vi "ReadFits-ExtractROI.vi"() -> ()   [LabVIEW 2011]
uses:
  <vilib>/Analysis/6fits.llb/Curve Fitting Criteria.ctl
  gfitsio/gfitsio-read-image-subset-i32-2d.vi
  Polymorphics/Distance(single).vi
  gfitsio/gfitsio.lvlib
  <vilib>/Analysis/NI_AALBase.lvlib
  <vilib>/Analysis/NI_AALPro.lvlib
panel:
  out "residue":dbl
  out "stdv":dbl
  out "amplitude":dbl
  out "center":dbl
  out "offset":dbl
  out "TmpData":i32[][](array[numeric])
  out "PSF X":dbl[](array[numeric])
  out "PSF Y":dbl[](array[numeric])
  in  "Use Barycen ?":bool
  out "XY Graph":cluster{"PSF X":dbl[], "PSF Y":dbl[]}[](graph)
  out "Cen Y":dbl
  out "Cen X":dbl
  out "ImageMedian":dbl format="%0.2f"
  out "Histogram Graph":T1(graph)
  in  "process":bool
  out "OutskirtMedian":dbl format="%0.2f"
  in  "save":bool
  in  "Length Y":i32
  in  "Length X":i32
  in  "Start Y":i32
  in  "Start X":i32
  out "ROI":i32[][](graph)
  out "Full Fits":i32[][](graph)
  in  "Path":path
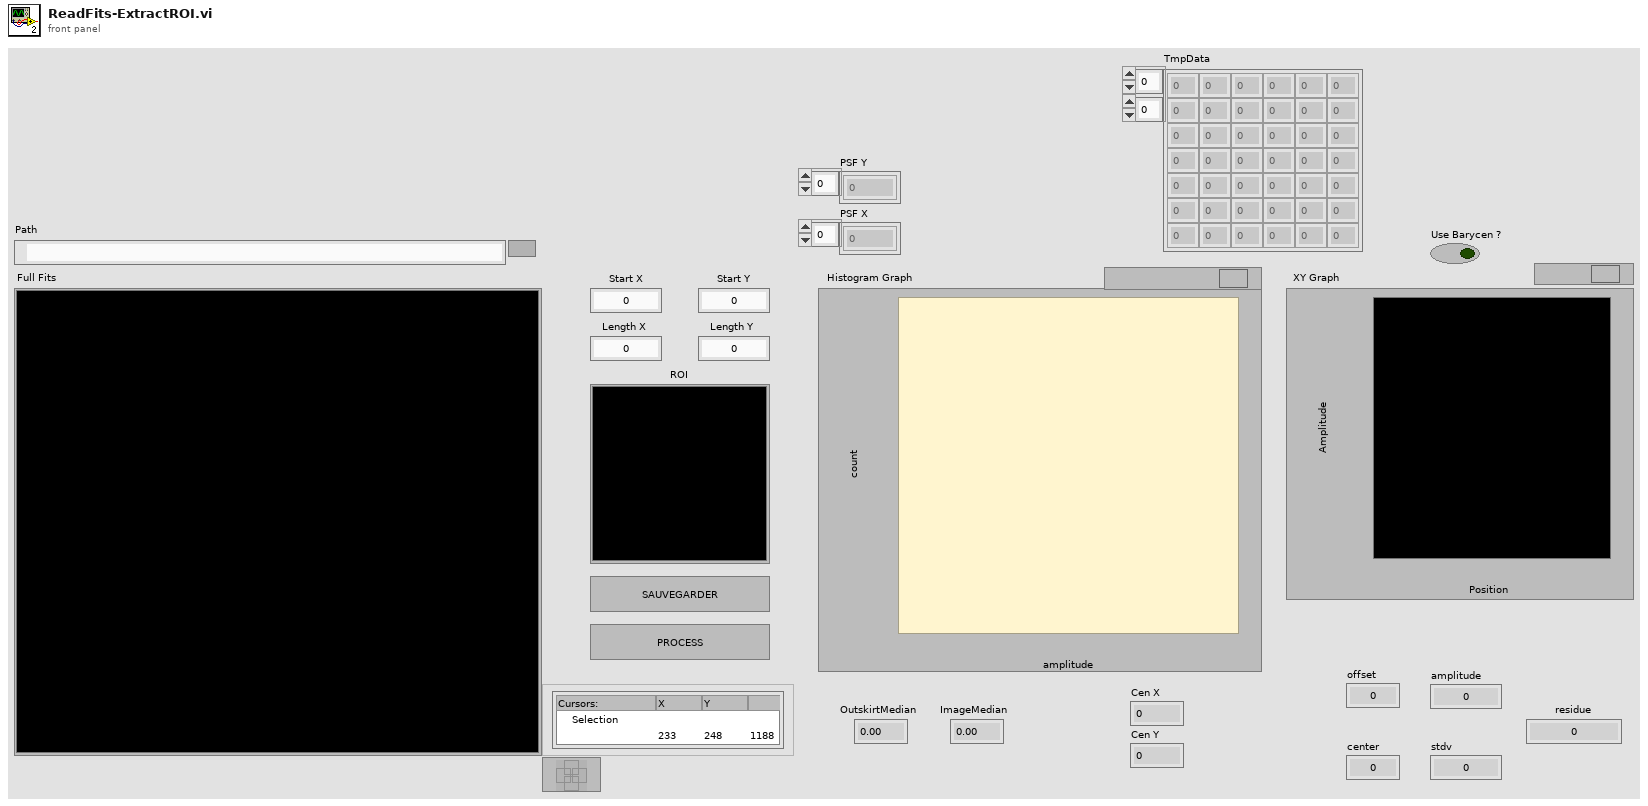
[diagram p1: front panel]
types:
  T1 = cluster{"X Values":dbl[], "Histogram: h(x)":i32[]}
  T2 = cluster{"amp min":dbl, "amp max":dbl, "center min":dbl, "center max":dbl, "deviation min":dbl, "deviation max":dbl, "offset min":dbl, "offset max":dbl}
  T3 = typedef "gfitsio.lvlib/gfitsio-refnum.ctl" = refnum<k1>
  T4 = typedef "NI_AALPro.lvlib/Curve Fitting Criteria.ctl" = u16
  T5 = cluster{dbl, "center min":dbl, "center min":dbl, "center min":dbl}
  T6 = cluster{"PSF X":dbl[], "Best Gaussian Fit":dbl[]}
  T7 = cluster{"PSF X":dbl[], "Best Gaussian Fit":dbl[]}[]
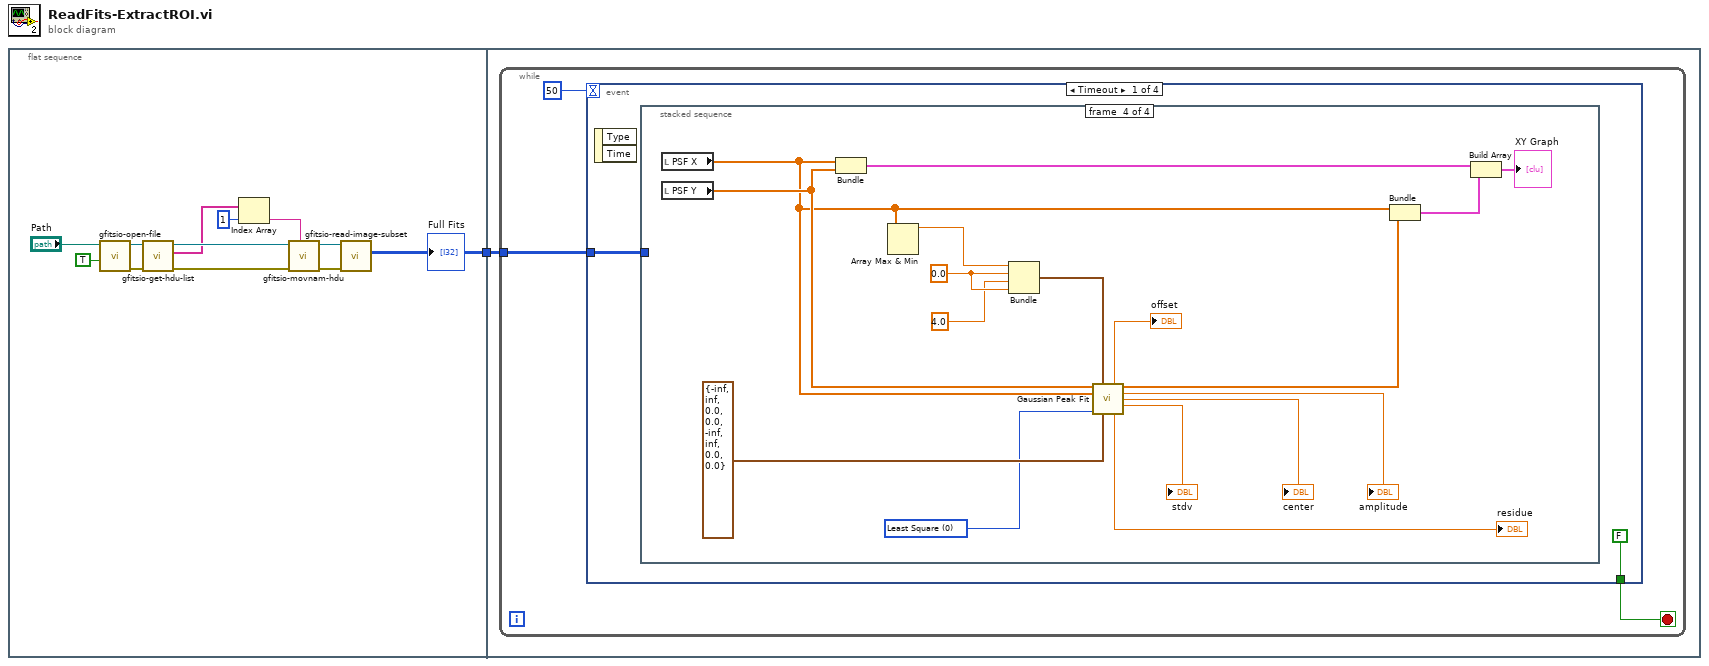
[diagram p0: block diagram]
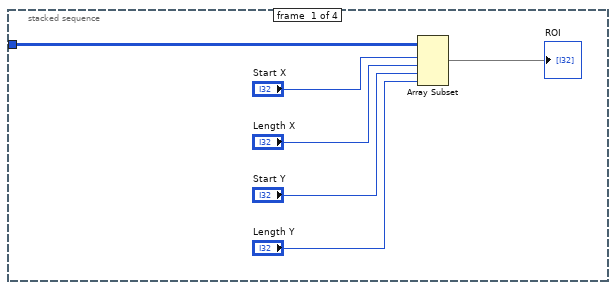
[diagram p2: hidden frame]
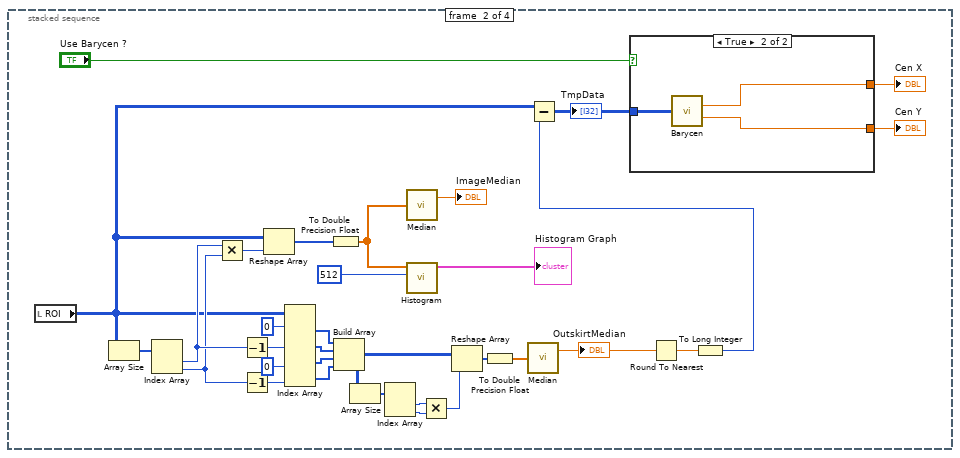
[diagram p3: hidden frame]
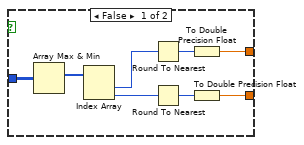
[diagram p4: hidden frame]
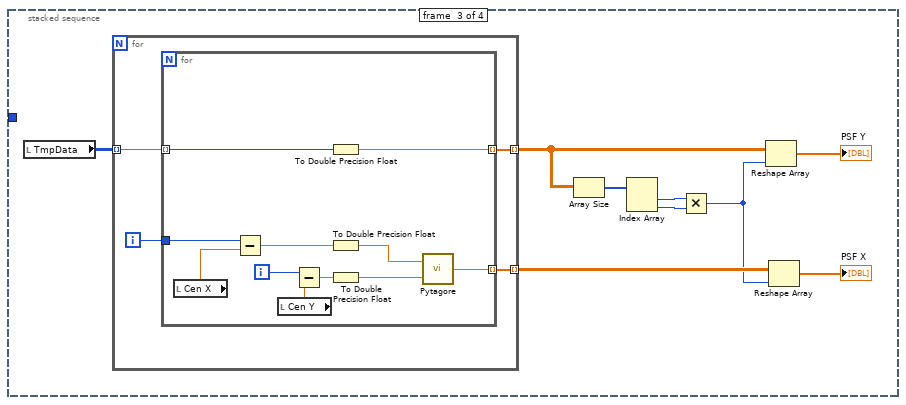
[diagram p5: hidden frame]
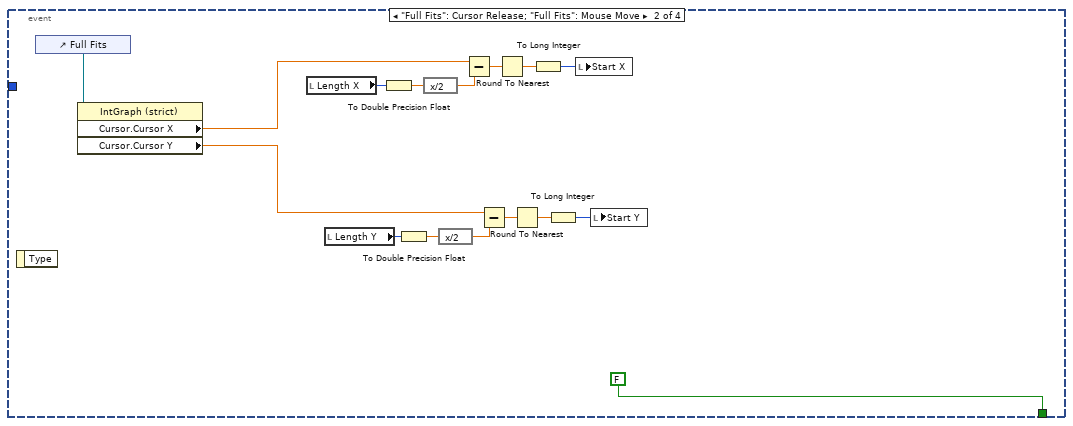
[diagram p6: hidden frame]
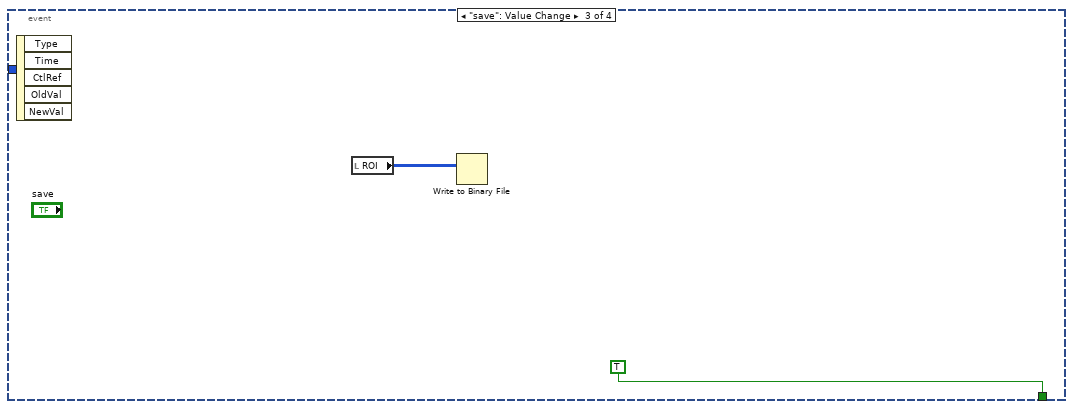
[diagram p7: hidden frame]
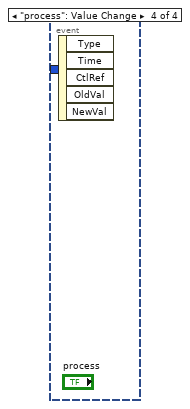
[diagram p8: hidden frame]
diagram:
  n1 = flat-sequence {
    tunnel: [w2] -> w1
    tunnel: w1 -> [w14]
    frame #0 {
      n2 = call "gfitsio-open-file.vi"("read only? (T:no)"=TRUE, "path"="Path") -> ("error out"=w6:errorcluster, "gfits refnum"=w7:T3)  [unwired: 8 in]
      n3 = call "gfitsio-get-hdu-list.vi"("error in (no error)"=w6, "gfits refnum"=w7) -> ("error out"=w8:errorcluster, "hdu names"=w5:string[], "dup gfits refnum"=w9:T3)  [unwired: 6 in, 1 out]
      n4 = Index Array(array=w5, index=1) -> (element=w3:string)
      n5 = call "gfitsio-movnam-hdu.vi"("extname"=w3, "error in (no error)"=w8, "gfits refnum"=w9) -> ("error out"=w11:errorcluster, "dup gfits refnum"=w10:T3)  [unwired: 7 in]
      n6 = call-poly "gfitsio-read-image-subset.vi"("error in (no error)"=w11, "gfits refnum"=w10) -> ("data"=w2:i32[][])  [unwired: 6 in, 3 out]
      "Full Fits" <- w2
    }
    frame #1 {
      n7 = while {
        tunnel: w14 -> [w17]
        stop <- w15 stop-if-true
        n8 = event shown="[0] Timeout" {
          selector: _ -> [_ _ _ _]
          dyn-events: _ -> [_ _ _ _]
          timeout: 50 -> [_ _ _ _]
          tunnel: w17 -> [w19 _ _ _]
          tunnel: [FALSE FALSE TRUE _] -> w15
          event Timeout {
            n9 = event-data() -> ()  [unwired: 1 in, 2 out]
            n10 = stacked-sequence {
              tunnel: w19 -> [w25 _ _ _]
              frame #0 {
                n11 = Array Subset(array=w25, index (row)="Start X", length (row)="Length X", index (col)="Start Y", length (col)="Length Y") -> (→"ROI":i32[][])
              }
              frame #1 {
                n12 = local read "ROI"() -> (w27:i32[][])
                n13 = Array Size(array=w27) -> (size(s)=w57:i32[])
                n14 = Index Array(array=w57) -> (element #1=w40:i32, element #2=w39:i32)  [unwired: 2 in]
                n15 = Multiply(x=w40, y=w39) -> (x*y=w41:i32)
                n16 = Decrement(x=w40) -> (x-1=w55:i32)
                n17 = Decrement(x=w39) -> (x-1=w54:i32)
                n18 = Reshape Array(w27, w41) -> (w38:i32[])
                n19 = Index Array(array=w27, index (row) #1=0, index (row) #2=w55, index (col) #3=0, index (col) #4=w54) -> (element #1=w49:i32[], element #2=w50:i32[], element #3=w51:i32[], element #4=w52:i32[])  [unwired: 4 in]
                n20 = To Double Precision Float(number=w38) -> (double precision float=w34:dbl[])
                n21 = Build Array(w49, w50, w51, w52) -> (w45:i32[][])
                n22 = Array Size(array=w45) -> (size(s)=w48:i32[])
                n23 = Index Array(array=w48) -> (element #1=w47:i32, element #2=w46:i32)  [unwired: 2 in]
                n24 = call <vilib>:"Median.vi"("X"=w34) -> ("median"=→"ImageMedian":dbl)  [unwired: 1 out]
                n25 = call <vilib>:"Histogram.vi"("intervals"=512, "X"=w34) -> ("Histogram Graph"=→"Histogram Graph":T1)  [unwired: 6 in, 3 out]
                n26 = Multiply(x=w47, y=w46) -> (x*y=w44:i32)
                n27 = Reshape Array(w45, w44) -> (w43:i32[])
                n28 = To Double Precision Float(number=w43) -> (double precision float=w42:dbl[])
                n29 = call <vilib>:"Median.vi"("X"=w42) -> ("median"=w29:dbl)  [unwired: 1 out]
                "OutskirtMedian" <- w29
                n30 = Round To Nearest(number=w29) -> (nearest integer value=w30:dbl)
                n31 = To Long Integer(number=w30) -> (32bit integer=w28:i32)
                n32 = Subtract(x=w27, y=w28) -> (x-y=w26:i32[][])
                "TmpData" <- w26
                n33 = case shown="True" "Use Barycen ?" {
                  tunnel: w26 -> [w65 w66]
                  tunnel: [w63 w68] -> w33
                  tunnel: [w59 w67] -> w32
                  frame False {
                    n34 = Array Max & Min(array=w65) -> (max index (indices)=w64:i32[])  [unwired: 3 out]
                    n35 = Index Array(array=w64) -> (element #1=w61:i32, element #2=w58:i32)  [unwired: 2 in]
                    n36 = Round To Nearest(number=w61) -> (nearest integer value=w62:i32)
                    n37 = Round To Nearest(number=w58) -> (nearest integer value=w60:i32)
                    n38 = To Double Precision Float(number=w62) -> (double precision float=w63:dbl)
                    n39 = To Double Precision Float(number=w60) -> (double precision float=w59:dbl)
                  }
                  frame True {
                    n40 = call "Barycen.vi"("Array"=w66) -> ("X?"=w68:dbl, "Y?"=w67:dbl)  [unwired: 13 in]
                  }
                }
                "Cen X" <- w33
                "Cen Y" <- w32
              }
              frame #2 {
                n41 = local read "TmpData"() -> (w69:i32[][])
                n42 = for {
                  tunnel: w69 -> [w81] mode=indexing
                  tunnel: [w79] -> w77 mode=indexing
                  tunnel: [w78] -> w76 mode=indexing
                  i -> [w80]
                  n43 = for {
                    tunnel: w81 -> [w83] mode=indexing
                    tunnel: w80 -> [w92]
                    tunnel: [w84] -> w79 mode=indexing
                    tunnel: [w82] -> w78 mode=indexing
                    i -> [w90]
                    n44 = local read "Cen X"() -> (w91:dbl)
                    n45 = Subtract(x=w92, y=w91) -> (x-y=w88:dbl)
                    n46 = local read "Cen Y"() -> (w89:dbl)
                    n47 = Subtract(x=w90, y=w89) -> (x-y=w87:dbl)
                    n48 = To Double Precision Float(number=w83) -> (double precision float=w82:dbl)
                    n49 = To Double Precision Float(number=w88) -> (double precision float=w86:dbl)
                    n50 = To Double Precision Float(number=w87) -> (double precision float=w85:dbl)
                    n51 = call-poly "Pytagore.vi"("D2"=w85, "D1"=w86) -> ("DT"=w84:dbl)
                  }
                }
                n52 = Array Size(array=w76) -> (size(s)=w75:i32[])
                n53 = Index Array(array=w75) -> (element #1=w74:i32, element #2=w73:i32)  [unwired: 2 in]
                n54 = Multiply(x=w74, y=w73) -> (x*y=w72:i32)
                n55 = Reshape Array(w76, w72) -> (→"PSF Y":dbl[])
                n56 = Reshape Array(w77, w72) -> (→"PSF X":dbl[])
              }
              frame #3 {
                w94 = T4 0 items=["Least Square", "Least Absolute Residual", "Bisquare"] ("method")
                w99 = 0.0 ("center min")
                n57 = local read "PSF X"() -> (w101:dbl[])
                n58 = local read "PSF Y"() -> (w106:dbl[])
                n59 = Bundle("PSF X"=w101, "PSF Y"=w106) -> (w108:cluster{"PSF X":dbl[], "PSF Y":dbl[]})  [unwired: 1 in]
                n60 = Array Max & Min(array=w101) -> (max value=w100:dbl)  [unwired: 3 out]
                n61 = Bundle(w100, "center min"=w99, "center min"=4.0, "center min"=w99) -> (w95:T5)  [unwired: 1 in]
                n62 = call <vilib>:"Gaussian Peak Fit.vi"("Y"=w106, "initial guess"=w95, "X"=w101, "method"=w94, "parameter bounds"=T2 {"amp min"=-inf, "amp max"=inf, "center min"=0.0, "center max"=0.0, "deviation min"=-inf, "deviation max"=inf, "offset min"=0.0, "offset max"=0.0}) -> ("offset"=→"offset":dbl, "Best Gaussian Fit"=w105:dbl[], "amplitude"=→"amplitude":dbl, "center"=→"center":dbl, "standard deviation"=→"stdv":dbl, "residue"=→"residue":dbl)  [unwired: 4 in, 1 out]
                n63 = Bundle("PSF X"=w101, "Best Gaussian Fit"=w105) -> (w109:T6)  [unwired: 1 in]
                n64 = Build Array(w108, w109) -> (→"XY Graph":T7)
              }
            }
          }
          event "Full Fits": Cursor Release; "Full Fits": Mouse Move {
            n65 = event-data() -> ()  [unwired: 1 in, 1 out]
            n66 = control-ref of="Full Fits"() -> (w112:refnum<vi>)
            n67 = property class="IntGraph (strict)"(reference=w112) -> ("Cursor.Cursor X"=w111:dbl, "Cursor.Cursor Y"=w110:dbl)  [unwired: 1 in, 2 out]
            n68 = local read "Length X"() -> (w113:i32)
            n69 = local read "Length Y"() -> (w121:i32)
            n70 = To Double Precision Float(number=w113) -> (double precision float=w117:dbl)
            n71 = To Double Precision Float(number=w121) -> (double precision float=w123:dbl)
            n72 = expression code="x/2"(w117) -> (w115:dbl)
            n73 = expression code="x/2"(w123) -> (w125:dbl)
            n74 = Subtract(x=w111, y=w115) -> (x-y=w116:dbl)
            n75 = Subtract(x=w110, y=w125) -> (x-y=w124:dbl)
            n76 = Round To Nearest(number=w116) -> (nearest integer value=w118:dbl)
            n77 = Round To Nearest(number=w124) -> (nearest integer value=w122:dbl)
            n78 = To Long Integer(number=w118) -> (32bit integer=w114:i32)
            n79 = To Long Integer(number=w122) -> (32bit integer=w120:i32)
            n80 = local write "Start X"(w114) -> ()
            n81 = local write "Start Y"(w120) -> ()
          }
          event "save": Value Change {
            n82 = event-data() -> ()  [unwired: 1 in, 5 out]
            n83 = local read "ROI"() -> (w126:i32[][])
            n84 = Write to Binary File(data=w126) -> ()  [unwired: 5 in, 3 out]
          }
          event "process": Value Change {
            n85 = event-data() -> ()  [unwired: 1 in, 5 out]
          }
        }
      }
    }
  }
